vi "IntensityScales_v2.vi"(4 "y\narray [T]\nstart/end [F]":bool, 5 "IntensityGraph in":refnum<vi>, 6 "x\narray [T]\nstart/end [F]":bool, 7 "Data":dbl[][](array[numeric]), 8 "y start & end":cluster{"y start":dbl, "y end":dbl}, 9 "Y Scale":dbl[](array[numeric]), 10 "x start & end":cluster{"x start":dbl, "x end":dbl}, 11 "X Scale":dbl[](array[numeric])) -> ()   [LabVIEW 2013]
uses:
  <vilib>/Utility/miscctls.llb/LVOffsetAndMultiplierTypeDef.ctl
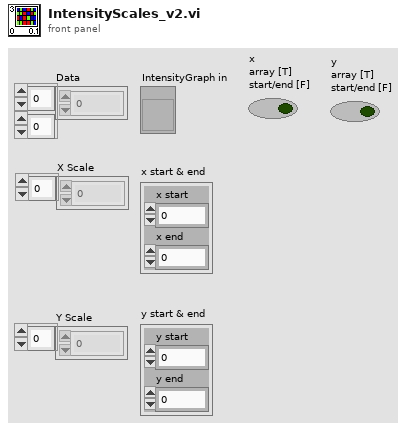
[diagram p1: front panel]
types:
  T1 = typedef "LVOffsetAndMultiplierTypeDef.ctl" = cluster{"Offset":dbl, "Multiplier":dbl}
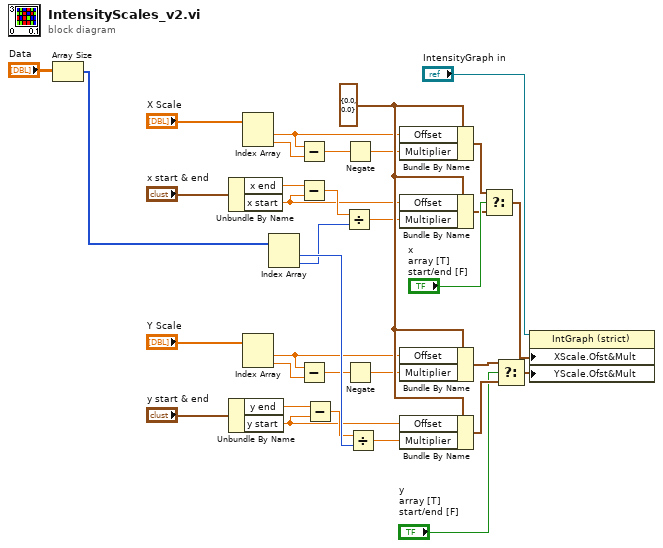
[diagram p0: block diagram]
diagram:
  w28 = T1 {"Offset"=0.0, "Multiplier"=0.0} ("X Scale.Offset and Multiplier")
  n1 = Array Size(array="Data") -> (size(s)=w20:i32[])
  n2 = Unbundle By Name("x start & end") -> ("x end"=w5:dbl, "x start"=w6:dbl)
  n3 = Unbundle By Name("y start & end") -> ("y end"=w3:dbl, "y start"=w2:dbl)
  n4 = Index Array(array="X Scale") -> (element #1=w11:dbl, element #2=w16:dbl)  [unwired: 2 in]
  n5 = Index Array(array="Y Scale") -> (element #1=w9:dbl, element #2=w13:dbl)  [unwired: 2 in]
  n6 = Index Array(array=w20) -> (element #1=w32:i32, element #2=w31:i32)  [unwired: 2 in]
  n7 = Subtract(x=w11, y=w16) -> (x-y=w15:dbl)
  n8 = Subtract(x=w5, y=w6) -> (x-y=w22:dbl)
  n9 = Subtract(x=w9, y=w13) -> (x-y=w14:dbl)
  n10 = Subtract(x=w3, y=w2) -> (x-y=w21:dbl)
  n11 = Divide(x=w22, y=w31) -> (x/y=w23:dbl)
  n12 = Negate(x=w15) -> (-x=w12:dbl)
  n13 = Negate(x=w14) -> (-x=w10:dbl)
  n14 = Divide(x=w21, y=w32) -> (x/y=w24:dbl)
  n15 = Bundle By Name(cluster=w28, "Offset"=w11, "Multiplier"=w12) -> (w29:T1)
  n16 = Bundle By Name(cluster=w28, "Offset"=w6, "Multiplier"=w23) -> (w26:T1)
  n17 = Bundle By Name(cluster=w28, "Offset"=w9, "Multiplier"=w10) -> (w25:T1)
  n18 = Bundle By Name(cluster=w28, "Offset"=w2, "Multiplier"=w24) -> (w27:T1)
  n19 = Select(t=w29, s="x\narray [T]\nstart/end [F]", f=w26) -> (s? t:f=w33:T1)
  n20 = Select(t=w25, s="y\narray [T]\nstart/end [F]", f=w27) -> (s? t:f=w34:T1)
  n21 = property on="Property Node" class="IntGraph (strict)"(reference="IntensityGraph in", "XScale.Ofst&Mult"=w33, "YScale.Ofst&Mult"=w34) -> ()  [unwired: 1 in, 2 out]
